vi "Insert Text.vi"(1 "Insert String":string, 2 "Insert Position":u32, 3 "Source String":string) -> (0 "Output String":string)   [LabVIEW 2023]
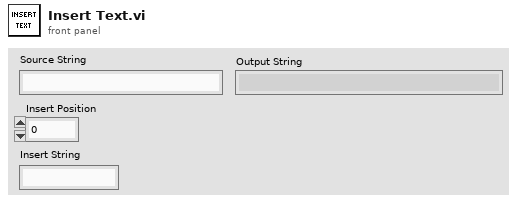
[diagram p1: front panel]
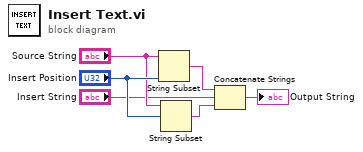
[diagram p0: block diagram]
diagram:
  n1 = String Subset(string="Source String", length (rest)="Insert Position") -> (substring=w4:string)  [unwired: 1 in]
  n2 = String Subset(string="Source String", offset (0)="Insert Position") -> (substring=w2:string)  [unwired: 1 in]
  n3 = Concatenate Strings(w4, "Insert String", w2) -> (→"Output String":string)
